vi "counter 2.vi"() -> ()   [LabVIEW 2010]
panel:
  out "전체 카운트":i32
  out "카운트 2":i32
  out "진행 중 합계":i32
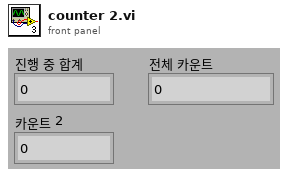
[diagram p1: front panel]
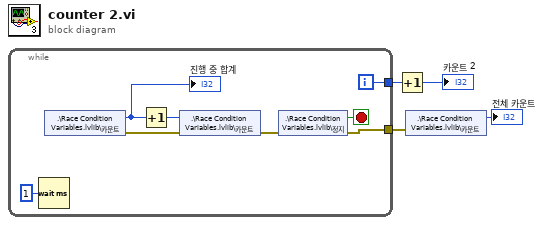
[diagram p0: block diagram]
diagram:
  n1 = while {
    tunnel: [w10] -> w4
    tunnel: [w9] -> w1
    i -> [w10]
    stop <- w5 stop-if-true
    n2 = Wait (ms)(milliseconds to wait=u32 1) -> ()  [unwired: 1 out]
    n3 = shared-variable ".\\Race Condition Variables.lvlib\\카운트"() -> (w6:i32, error out=w12:errorcluster)  [unwired: 1 in]
    "진행 중 합계" <- w6
    n4 = Increment(x=w6) -> (x+1=w7:i32)
    n5 = shared-variable ".\\Race Condition Variables.lvlib\\카운트"(w7, error in=w12) -> (error out=w11:errorcluster)
    n6 = shared-variable ".\\Race Condition Variables.lvlib\\정지"(error in=w11) -> (w5:bool, error out=w9:errorcluster)
  }
  n7 = Increment(x=w4) -> (x+1=→"카운트 2":i32)
  n8 = shared-variable ".\\Race Condition Variables.lvlib\\카운트"(error in=w1) -> (→"전체 카운트":i32)  [unwired: 1 out]
